vi "Event Text For Register.vi"(8 "hotel":string, 9 "guest":string, 10 "first registration?":bool, 11 "already registered?":bool) -> (3 "message":string)   [LabVIEW 2023]
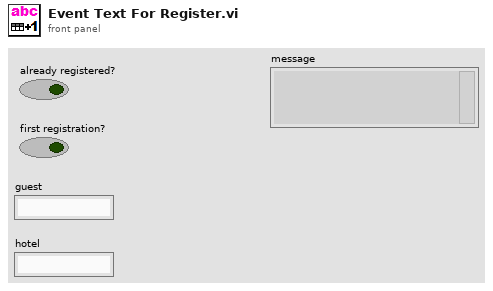
[diagram p1: front panel]
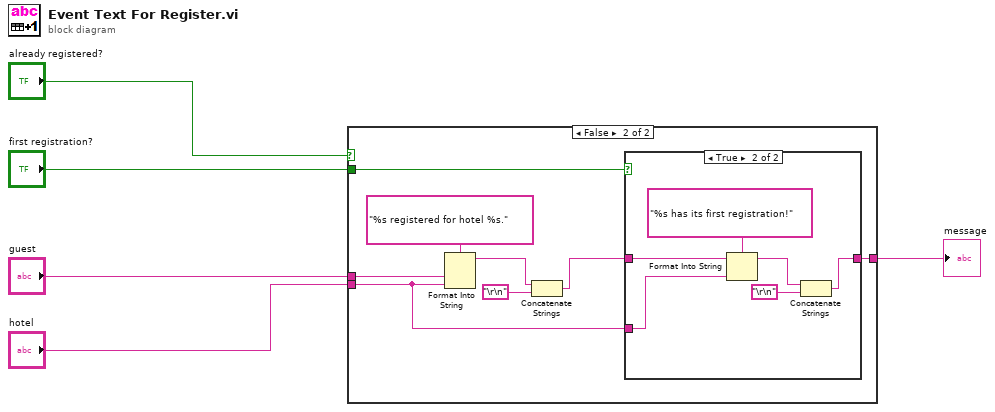
[diagram p0: block diagram]
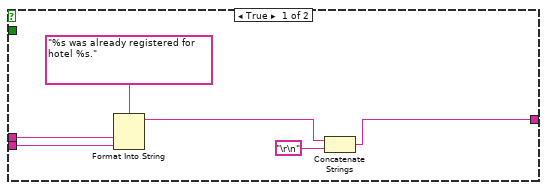
[diagram p2: hidden frame]
diagram:
  n1 = case shown="False" "already registered?" {
    tunnel: "guest" -> [w10 w18]
    tunnel: "hotel" -> [w9 w12]
    tunnel: [w6 w16] -> w4
    tunnel: "first registration?" -> [_ w17]
    frame True {
      n2 = Format Into String(format string="%s was already registered for hotel %s." ("L10n_message 1"), w10, w9) -> (resulting string=w7:string)  [unwired: 2 in, 1 out]
      n3 = Concatenate Strings(w7, "\r\n") -> (w6:string)
    }
    frame False {
      n4 = Format Into String(format string="%s registered for hotel %s." ("L10n_message 2"), w18, w12) -> (resulting string=w15:string)  [unwired: 2 in, 1 out]
      n5 = Concatenate Strings(w15, "\r\n") -> (w13:string)
      n6 = case shown="True" w17 {
        tunnel: w13 -> [w20 w25]
        tunnel: [w20 w22] -> w16
        tunnel: w12 -> [_ w21]
        frame False {
        }
        frame True {
          n7 = Format Into String(format string="%s has its first registration!" ("L10n_message 3"), initial string=w25, w21) -> (resulting string=w23:string)  [unwired: 1 in, 1 out]
          n8 = Concatenate Strings(w23, "\r\n") -> (w22:string)
        }
      }
    }
  }
  "message" <- w4
